vi "readData.vi"(8 "error in (no error)":errorcluster, 10 "array":string[][](array[string]), 11 "DDSFileReader in":refnum<class "DDSFileReader.lvclass">) -> (0 "error out":errorcluster, 1 "Array":dbl[][](array[numeric]), 2 "channels":string, 3 "DDSFileReader out":refnum<class "DDSFileReader.lvclass">, 4 "Defaults":dbl[](array[numeric]), 5 "channelAddresses":string[](array[string]))   [LabVIEW 2011, in "Tools.lvlib" / "Filing.lvlib" / "DDSFileReader.lvclass"]
uses:
  DDSFileReader.lvclass
  DDSFileReader.lvclass/DDSFileReader.ctl
panel:
  out "Array 2":dbl[][](array[numeric])
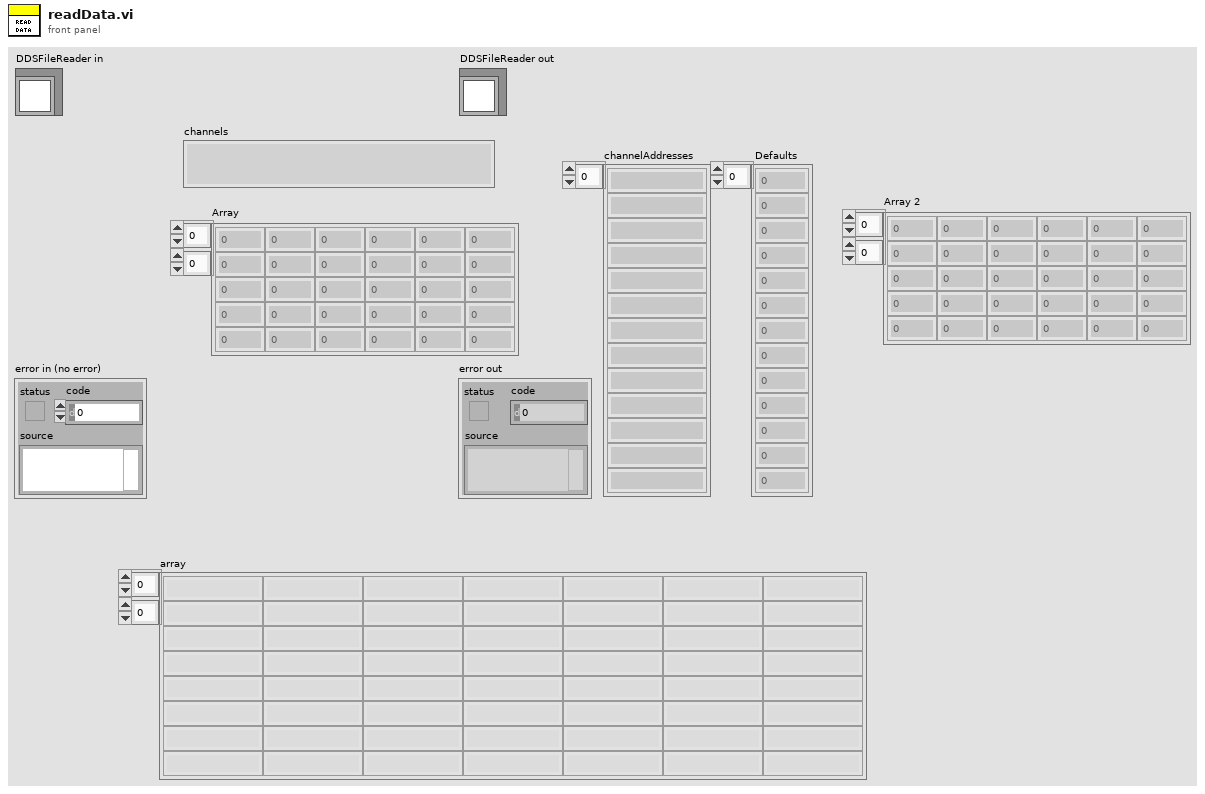
[diagram p1: front panel]
types:
  T1 = cluster{"data (time, freq, amplitude, phase)":dbl[][]}
  T2 = cluster{"Frequency(MHz)":dbl, "Amplitude":dbl, "Phase":dbl, "OutputForm":enum16{"Sine", "Square", "Triangle", "Arbitrary"}}
  T3 = cluster{"Frequency(MHz)":dbl, "Amplitude":dbl, "Phase":dbl, "OutputForm":enum16{"Sine", "Square", "Triangle", "Arbitrary"}}[]
  T4 = cluster{"data (time, freq, amplitude, phase)":dbl[][]}[]
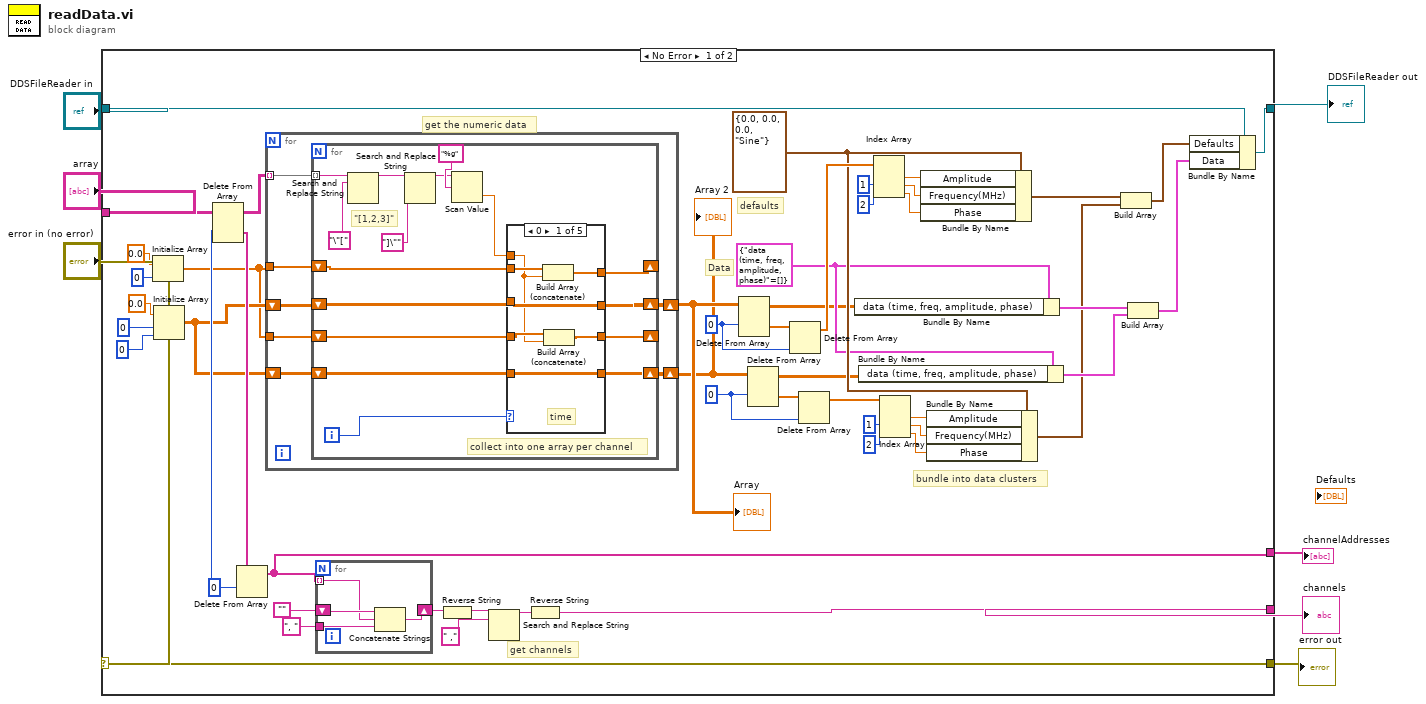
[diagram p0: block diagram]
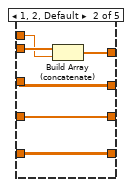
[diagram p2: hidden frame]
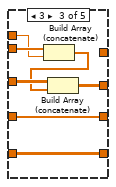
[diagram p3: hidden frame]
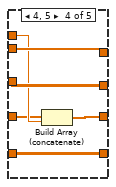
[diagram p4: hidden frame]
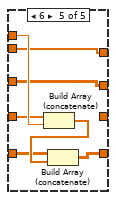
[diagram p5: hidden frame]
diagram:
  n1 = case shown="No Error" "error in (no error)" {
    selector: "error in (no error)" -> [w57 w119]
    tunnel: [w57 w119] -> w4
    tunnel: [w18 w118] -> w6
    tunnel: "DDSFileReader in" -> [w21 w118]
    tunnel: "array" -> [w48 _]
    tunnel: [w46 _] -> w2
    tunnel: [w45 _] -> w3
    frame No Error {
      w27 = T1 {"data (time, freq, amplitude, phase)"=[]} ("Sequence")
      w28 = T2 {"Frequency(MHz)"=0.0, "Amplitude"=0.0, "Phase"=0.0, "OutputForm"=enum."Sine"} ("OutputDefaults")
      w41 = 0 ("index (row)")
      w43 = 0 ("index (row)")
      w47 = 0 ("index")
      # "Data"
      # "defaults"
      # "bundle into data clusters"
      # "get channels"
      # "get the numeric data"
      n2 = Initialize Array(0.0 ("element"), 0 ("dimension size")) -> (w10:dbl[])
      n3 = Initialize Array(0.0 ("element"), 0 ("dimension size"), 0 ("dimension size")) -> (w11:dbl[][])
      n4 = Delete From Array(array=w48, index (row)=w47) -> (deleted portion=w51:string[], array with subset deleted=w50:string[][])  [unwired: 2 in]
      n5 = Delete From Array(array=w51, index=w47) -> (array with subset deleted=w45:string[])  [unwired: 1 in, 1 out]
      n6 = for {
        tunnel: w50 -> [w64] mode=indexing
        shift-right: [w63] -> w9
        shift-left: w11 -> [w62]
        shift-right: [w61] -> w8
        shift-left: w11 -> [w60]
        tunnel: w10 -> [w59]
        tunnel: w10 -> [w58]
        n7 = for {
          tunnel: w64 -> [w79] mode=indexing
          shift-right: [w71] -> _
          shift-left: w59 -> [w72]
          shift-right: [w70] -> w63
          shift-left: w62 -> [w69]
          shift-right: [w68] -> _
          shift-left: w58 -> [w67]
          shift-right: [w66] -> w61
          shift-left: w60 -> [w65]
          i -> [w74]
          # "collect into one array per channel"
          # "\"[1,2,3]\""
          n8 = Search and Replace String(input string=w79, search string="\"[") -> (result string=w78:string)  [unwired: 6 in, 3 out]
          n9 = Search and Replace String(input string=w78, search string="]\"") -> (result string=w75:string)  [unwired: 6 in, 3 out]
          n10 = Scan Value(string=w75, format string="%g") -> (value=w73:dbl)  [unwired: 1 in, 1 out]
          n11 = case shown="0" w74 {
            tunnel: w73 -> [w81 w91 w99 w104 w113]
            tunnel: w72 -> [w87 w93 w100 w105 w110]
            tunnel: [w86 w92 _ w105 w110] -> w71
            tunnel: [w85 w90 w98 w106 w109] -> w70
            tunnel: w69 -> [w85 w90 w97 w106 w109]
            tunnel: [w83 w89 w95 w103 _] -> w68
            tunnel: w67 -> [w82 w89 w95 w102 w111]
            tunnel: [w84 w88 w94 w101 w108] -> w66
            tunnel: w65 -> [w84 w88 w94 w101 w107]
            frame 0 {
              # "time"
              n12 = Build Array (concatenate)(w87, w81) -> (w86:dbl[])
              n13 = Build Array (concatenate)(w82, w81) -> (w83:dbl[])
            }
            frame 1, 2, Default {
              n14 = Build Array (concatenate)(w93, w91) -> (w92:dbl[])
            }
            frame 3 {
              n15 = Build Array (concatenate)(w100, w99) -> (w96:dbl[])
              n16 = Build Array (concatenate)(w97, w96) -> (w98:dbl[][])
            }
            frame 4, 5 {
              n17 = Build Array (concatenate)(w102, w104) -> (w103:dbl[])
            }
            frame 6 {
              n18 = Build Array (concatenate)(w111, w113) -> (w112:dbl[])
              n19 = Build Array (concatenate)(w107, w112) -> (w108:dbl[][])
            }
          }
        }
      }
      "Array" <- w9
      "Array 2" <- w8
      n20 = for {
        tunnel: w45 -> [w116] mode=indexing
        shift-right: [w115] -> w55
        shift-left: "" -> [w117]
        tunnel: ", " -> [w114]
        n21 = Concatenate Strings(w117, w116, w114) -> (w115:string)
      }
      n22 = Reverse String(1:w55) -> (0:w54:string)
      n23 = Search and Replace String(input string=w54, search string=" ,") -> (result string=w52:string)  [unwired: 6 in, 3 out]
      n24 = Reverse String(1:w52) -> (0:w46:string)
      n25 = Delete From Array(array=w9, index (row)=w43) -> (deleted portion=w44:dbl[], array with subset deleted=w26:dbl[][])  [unwired: 2 in]
      n26 = Delete From Array(array=w8, index (row)=w41) -> (deleted portion=w42:dbl[], array with subset deleted=w17:dbl[][])  [unwired: 2 in]
      n27 = Delete From Array(array=w44, index=w43) -> (array with subset deleted=w40:dbl[])  [unwired: 1 in, 1 out]
      n28 = Delete From Array(array=w42, index=w41) -> (array with subset deleted=w29:dbl[])  [unwired: 1 in, 1 out]
      n29 = Bundle By Name(cluster=w27, "data (time, freq, amplitude, phase)"=w26) -> (w25:T1)
      n30 = Bundle By Name(cluster=w27, "data (time, freq, amplitude, phase)"=w17) -> (w24:T1)
      n31 = Index Array(array=w40, index #2=1, index #3=2 ("index")) -> (element #1=w39:dbl, element #2=w38:dbl, element #3=w37:dbl)  [unwired: 1 in]
      n32 = Index Array(array=w29, index #2=1, index #3=2 ("index")) -> (element #1=w34:dbl, element #2=w33:dbl, element #3=w32:dbl)  [unwired: 1 in]
      n33 = Bundle By Name(cluster=w28, "Amplitude"=w39, "Frequency(MHz)"=w38, "Phase"=w37) -> (w23:T2)
      n34 = Bundle By Name(cluster=w28, "Amplitude"=w34, "Frequency(MHz)"=w33, "Phase"=w32) -> (w22:T2)
      n35 = Build Array(w23, w22) -> (w20:T3)
      n36 = Build Array(w25, w24) -> (w19:T4)
      n37 = Bundle By Name(cluster=w21, "Defaults"=w20, "Data"=w19) -> (w18:refnum<class "DDSFileReader.lvclass">)
    }
    frame Error {
    }
  }
  "error out" <- w4
  "DDSFileReader out" <- w6
  "channels" <- w2
  "channelAddresses" <- w3
